vi "Run AliasVi.vi"(8 "error in (no error)":errorcluster caption="错误输入（无错误）", 10 "Vi Alias":string, 11 "PanelDataNode 输入":refnum<class "PanelDataNode.lvclass"> caption="DNL_LabVIEW Object in") -> (0 "error out":errorcluster caption="错误输出", 2 "VI*":refnum<vi>, 3 "PanelDataNode 输出":refnum<class "PanelDataNode.lvclass"> caption="DNL_LabVIEW Object out")   [LabVIEW 2016, in "PanelDataNode.lvclass"]
uses:
  PanelDataNode.lvclass
  PanelDataNode.lvclass/PanelDataNode.ctl
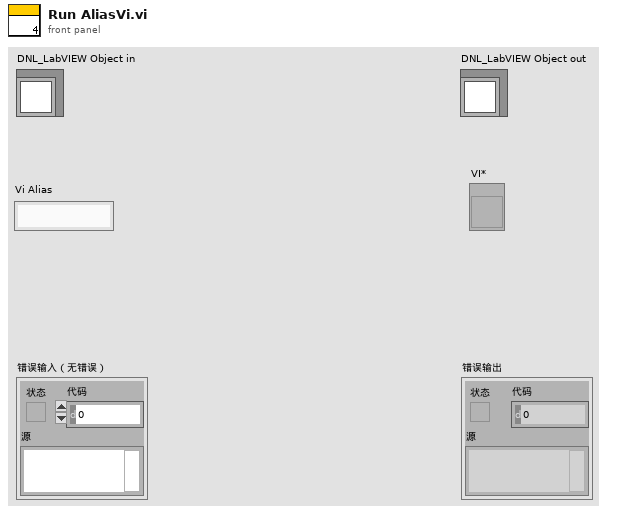
[diagram p1: front panel]
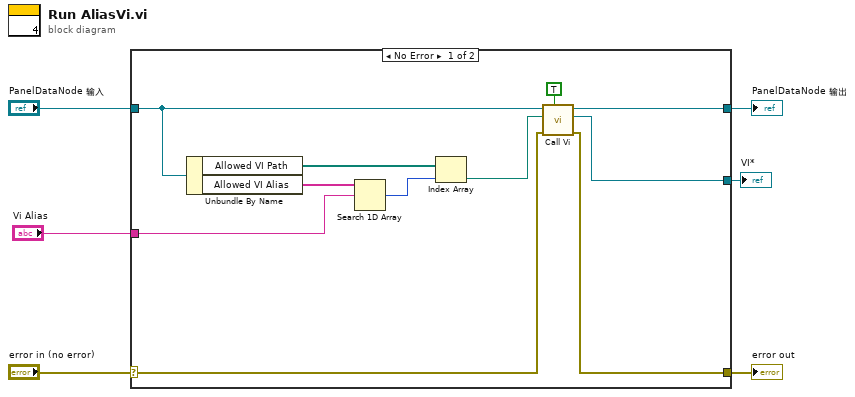
[diagram p0: block diagram]
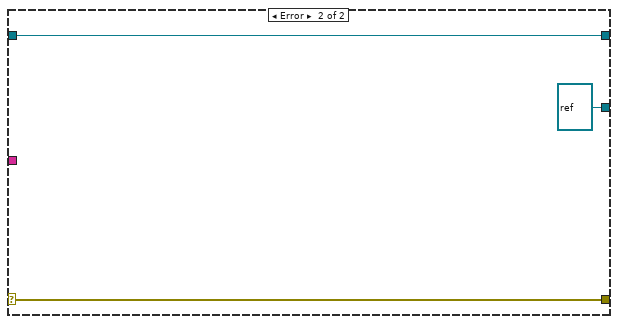
[diagram p2: hidden frame]
diagram:
  n1 = case shown="No Error" "error in (no error)" {
    selector: "error in (no error)" -> [w8 w20]
    tunnel: [w7 w20] -> w5
    tunnel: [w11 w19] -> w3
    tunnel: "PanelDataNode 输入" -> [w12 w19]
    tunnel: "Vi Alias" -> [w16 _]
    tunnel: [w10 refnum<vi> refnum ("VI*")] -> w1
    frame No Error {
      n2 = Unbundle By Name(w12) -> ("Allowed VI Path"=w15:path[], "Allowed VI Alias"=w17:string[])
      n3 = Search 1D Array(1D array=w17, element=w16) -> (index of element=w14:i32)  [unwired: 1 in]
      n4 = Index Array(array=w15, index=w14) -> (element=w13:path)
      n5 = call-dynamic "Call Vi.vi"("Auto Dispose Ref"=TRUE, "error in (no error)"=w8, "Vi Path"=w13, "PanelDataNode 输入"=w12) -> ("error out"=w7:errorcluster, "VI*"=w10:refnum<vi>, "PanelDataNode 输出"=w11:refnum<class "PanelDataNode.lvclass">)  [unwired: 5 in]
    }
    frame Error {
    }
  }
  "error out" <- w5
  "PanelDataNode 输出" <- w3
  "VI*" <- w1
